vi "GetType.vi"(8 "error in (no error)":errorcluster, 11 "Reset Min-Max Msg":refnum<class "Reset Min-Max Msg.lvclass">) -> (0 "error out":errorcluster, 2 "Data Sample":variant, 3 "Reset Min-Max Msg":refnum<class "Reset Min-Max Msg.lvclass">)   [LabVIEW 2016, in "LS218.lvlib" / "Reset Min-Max Msg.lvclass"]
uses:
  Reset Min-Max Msg.lvclass
  Reset Min-Max Msg.lvclass/Reset Min-Max Msg.ctl
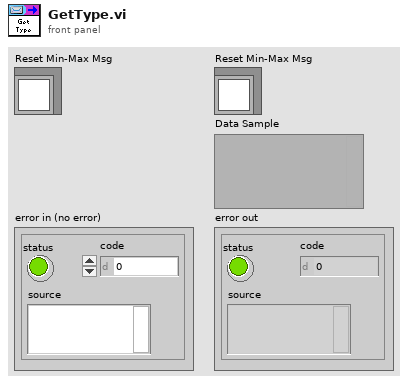
[diagram p1: front panel]
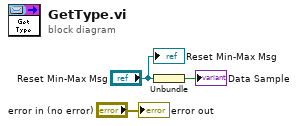
[diagram p0: block diagram]
diagram:
  n1 = Unbundle("Reset Min-Max Msg") -> (→"Data Sample":bool)
  "error out" <- "error in (no error)"
  "Reset Min-Max Msg" <- "Reset Min-Max Msg"
